vi "Read channel classification.vi"(8 "error in":errorcluster, 11 "channel in":refnum<class "TBM channel.lvclass">) -> (0 "error out":errorcluster, 2 "channel classification":T1, 3 "channel out":refnum<class "TBM channel.lvclass">)   [LabVIEW 2013, in "TBM channel.lvclass"]
doc: "Gets the classification/direction of a channel."
uses:
  TBM channel.lvclass
  channel classification.ctl
  TBM channel.lvclass/TBM channel.ctl
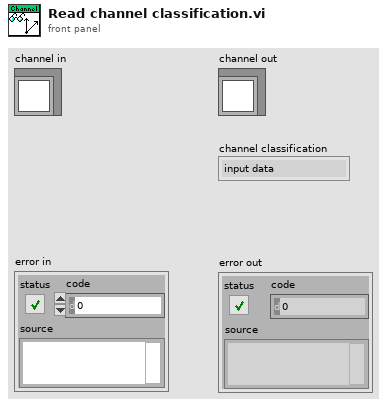
[diagram p1: front panel]
types:
  T1 = typedef "TBM channel.lvclass/channel classification.ctl" = enum16{"input data", "output data", "processing parameter", "processing result"}
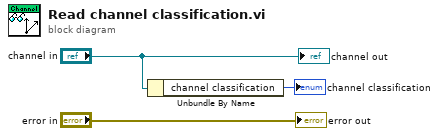
[diagram p0: block diagram]
diagram:
  n1 = Unbundle By Name("channel in") -> ("channel classification"=→"channel classification":T1)
  "channel out" <- "channel in"
  "error out" <- "error in"
